vi "LabViewDllTest (SubVI).vi"(9 "Array":dbl[](array[numeric]), 10 "c":dbl, 11 "Numeric":i32) -> (2 "a":dbl[](array[numeric]), 3 "return val":i32)   [LabVIEW 2017]
uses:
  x64/Release/LabViewDllTest.dll
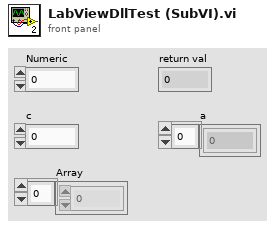
[diagram p1: front panel]
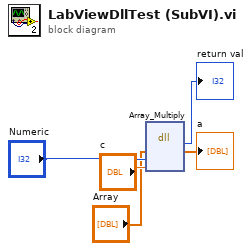
[diagram p0: block diagram]
diagram:
  n1 = dll-call lib="C:/Users/Paul/Documents/Visual Studio 2008/Projects/LabViewDllTest/x64/Release/LabViewDllTest.dll" fn="Array_Multiply"("a"="Array", "n"="Numeric", "c"="c") -> ("return val"=→"return val":i32, "a"=→"a":dbl[])  [unwired: 5 in, 2 out]
